vi "Extract TDMS DAQ Info.vi"(8 "error in (no error)":errorcluster, 10 "TDMS Name Mapping":T1, 11 "TDMS File Path":path) -> (0 "error out":errorcluster, 1 "DAQ Sample Rate":dbl, 2 "DAQ Wfm Map":map{string, digitalwaveform}(c390), 3 "DAQ Channels":string[](array[string]))   [LabVIEW 2025]
uses:
  Typedef/TDMS Name Mapping.ctl
  <vilib>/Utility/error.llb/Error Cluster From Error Code.vi
  <vilib>/Waveform/DWDTOps.llb/DWDT Boolean Array to Digital.vi
  <vilib>/ErrorRing/Error Ring.xnode
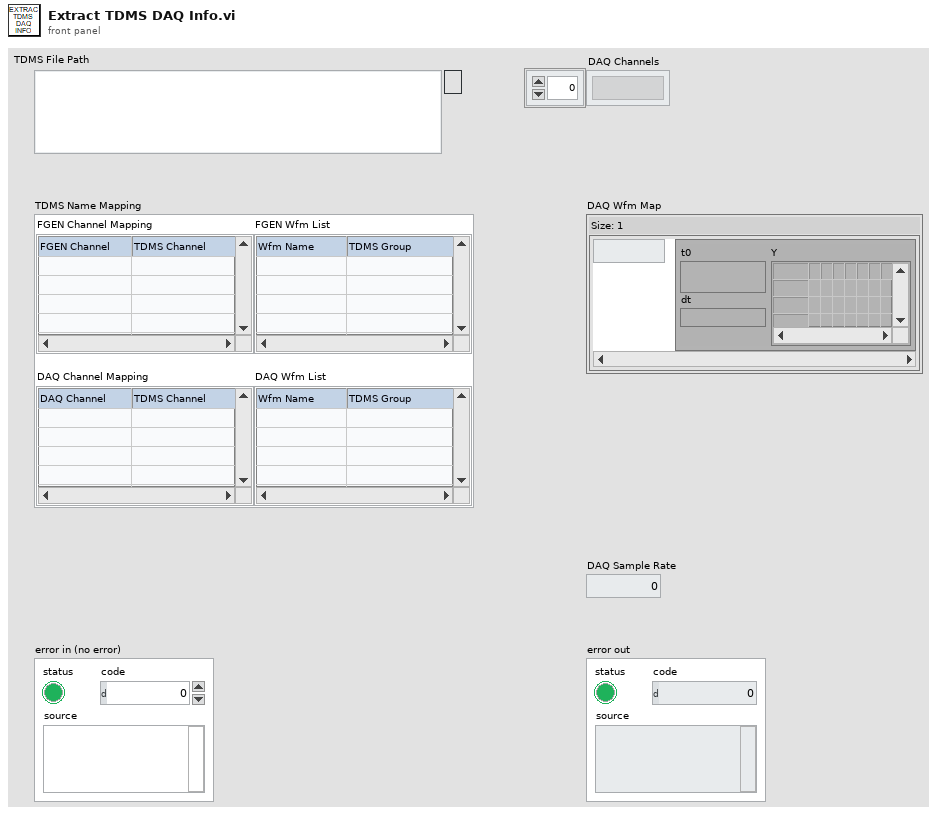
[diagram p1: front panel]
types:
  T1 = typedef "TDMS Name Mapping.ctl" = cluster{"FGEN Channel Mapping":string[][], "DAQ Channel Mapping":string[][], "FGEN Wfm List":string[][], "DAQ Wfm List":string[][]}
  T2 = enum16{"open", "open or create", "create or replace", "create", "open (read-only)"}
  T3 = enum16{"Error or Wfm Not Found", "Not all Chns Found", "All Found"}
  T4 = cluster{"Waveforms":waveform(dbl)[], "Markers":i32}
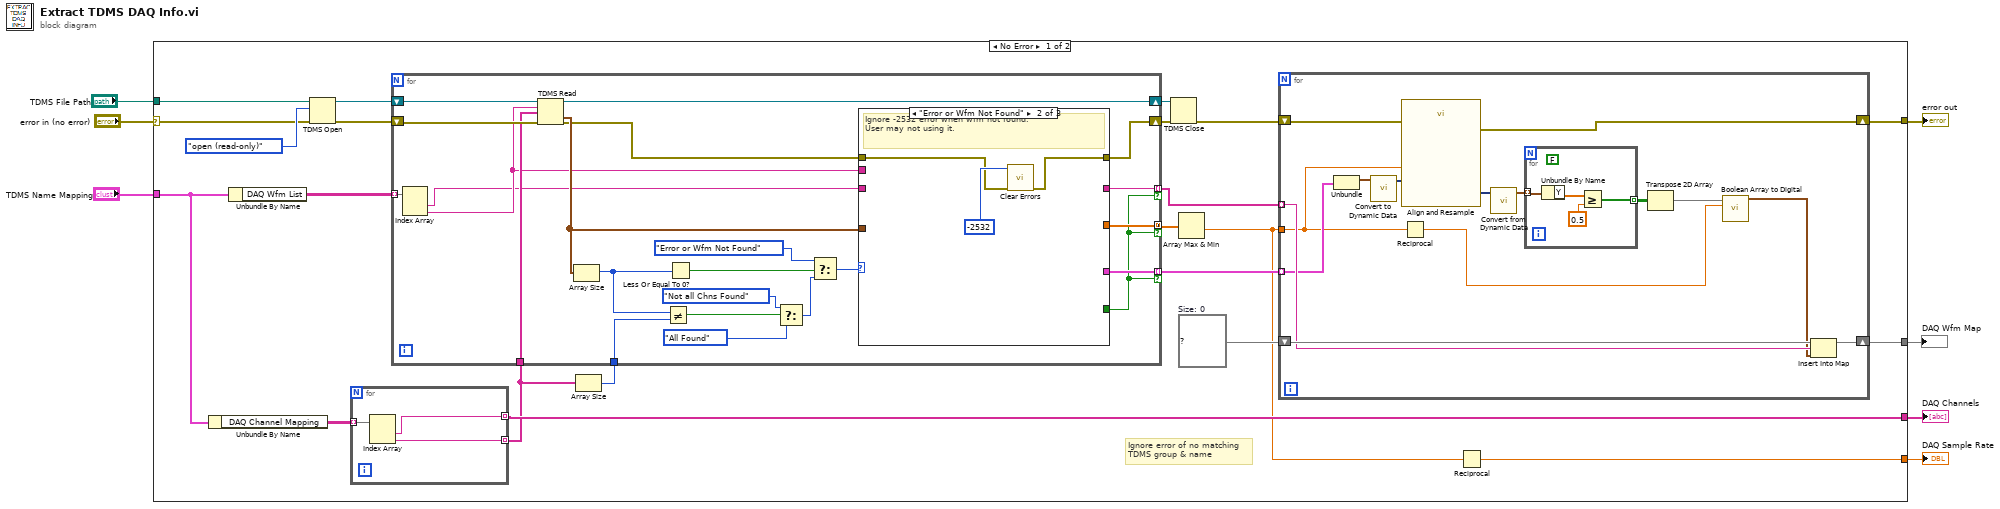
[diagram p0: block diagram]
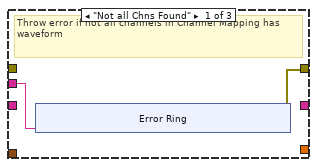
[diagram p2: hidden frame]
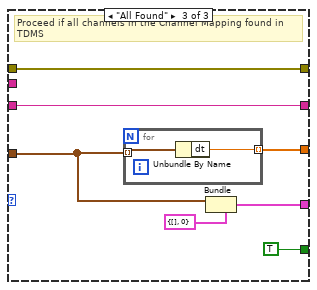
[diagram p3: hidden frame]
diagram:
  n1 = case shown="No Error" "error in (no error)" {
    selector: "error in (no error)" -> [w20 w96]
    tunnel: "TDMS File Path" -> [w27 _]
    tunnel: [w26 _] -> w6
    tunnel: [w14 w96] -> w5
    tunnel: [w13 _] -> w1
    tunnel: [w11 _] -> w3
    tunnel: "TDMS Name Mapping" -> [w10 _]
    frame No Error {
      w17 = map{string, digitalwaveform} {}  # Size: 0
      # "Ignore error of no matching\nTDMS group & name"
      n2 = Unbundle By Name(w10) -> ("DAQ Channel Mapping"=w28:string[][])
      n3 = Unbundle By Name(w10) -> ("DAQ Wfm List"=w29:string[][])
      n4 = TDMS Open(8:w20, 10:T2."open (read-only)" ("operation (0:open)"), 11:w27) -> (0:w24:errorcluster, 3:w25:refnum<k34>)  [unwired: 4 in]
      n5 = for {
        tunnel: w28 -> [w76] mode=indexing
        tunnel: [w75] -> w26 mode=indexing
        tunnel: [w74] -> w9 mode=indexing
        n6 = Index Array(array=w76) -> (element #1=w75:string, element #2=w74:string)  [unwired: 2 in]
      }
      n7 = Array Size(array=w9) -> (size(s)=w8:i32)
      n8 = for {
        tunnel: w29 -> [w52] mode=indexing
        tunnel: [w40] -> w15 mode=indexing if=w39
        tunnel: w9 -> [w46]
        shift-right: [w45] -> w21
        shift-left: w24 -> [w50]
        shift-right: [w49] -> w22
        shift-left: w25 -> [w51]
        tunnel: [w48] -> w18 mode=indexing if=w39
        tunnel: [w47] -> w19 mode=concatenating if=w39
        tunnel: w8 -> [w31]
        n9 = Index Array(array=w52) -> (element #1=w41:string, element #2=w42:string)  [unwired: 2 in]
        n10 = TDMS Read(0:w51, 5:w42, 7:w46, 11:w50) -> (4:w49:refnum<k34>, 10:w44:waveform(dbl)[], 15:w43:errorcluster)  [unwired: 4 in, 3 out]
        n11 = Array Size(array=w44) -> (size(s)=w32:i32)
        n12 = Not Equal?(x=w32, y=w31) -> (x != y?=w34:bool)
        n13 = Less Or Equal To 0?(x=w32) -> (x <= 0?=w37:bool)
        n14 = Select(t=T3."Not all Chns Found", s=w34, f=T3."All Found") -> (s? t:f=w35:T3)
        n15 = Select(t=T3."Error or Wfm Not Found", s=w37, f=w35) -> (s? t:f=w30:T3)
        n16 = case shown="\"Error or Wfm Not Found\"" w30 {
          tunnel: [_ _ w70] -> w48
          tunnel: w44 -> [_ _ w66]
          tunnel: [_ _ w69] -> w47
          tunnel: w43 -> [_ w63 w68]
          tunnel: [w53 w62 w68] -> w45
          tunnel: w42 -> [w54 _ _]
          tunnel: w41 -> [_ _ w67]
          tunnel: [_ _ w67] -> w40
          tunnel: [_ _ TRUE] -> w39
          frame "Not all Chns Found" {
            # "Throw error if not all channels in Channel Mapping has waveform"
            n17 = xnode "Error Ring"("parameter 0"=w54) -> ("error out"=w53:errorcluster)
          }
          frame "Error or Wfm Not Found" {
            # "Ignore -2532 error when wfm not found.\nUser may not using it."
            n18 = call <vilib>:"Clear Errors.vi"("error in (no error)"=w63, "specific error code to clear (0: all)"=-2532) -> ("error out"=w62:errorcluster)  [unwired: 4 in, 1 out]
          }
          frame "All Found" {
            # "Proceed if all channels in the Channel Mapping found in TDMS"
            n19 = for {
              tunnel: w66 -> [w73] mode=indexing
              tunnel: [w72] -> w69 mode=indexing
              n20 = Unbundle By Name(w73) -> ("dt"=w72:dbl)
            }
            n21 = Bundle(cluster=T4 {"Waveforms"=[], "Markers"=0} ("output cluster"), "Waveforms"=w66) -> (w70:T4)  [unwired: 1 in]
          }
        }
      }
      n22 = TDMS Close(8:w21, 11:w22) -> (0:w16:errorcluster)  [unwired: 1 out]
      n23 = Array Max & Min(array=w19) -> (min value=w12:dbl)  [unwired: 3 out]
      n24 = for {
        tunnel: w18 -> [w83] mode=indexing
        shift-right: [w90] -> w13
        shift-left: w17 -> [w91]
        tunnel: w12 -> [w81]
        shift-right: [w88] -> w14
        shift-left: w16 -> [w89]
        tunnel: w15 -> [w84] mode=indexing
        n25 = Unbundle(w83) -> ("Waveforms"=w87:waveform(dbl)[])  [unwired: 1 out]
        n26 = call "Convert to Dynamic Data"("Array of Waveforms"=w87) -> ("Dynamic Data Type"=w86:dynamicdata)  [unwired: 3 in]
        n27 = call "Align and Resample"("dt"=w81, "error in (no error)"=w89, "Signals"=w86) -> ("error out"=w88:errorcluster, "Resampled Signals"=w85:dynamicdata)  [unwired: 6 in, 1 out]
        n28 = Reciprocal(x=w81) -> (1/x=w80:dbl)
        n29 = call "Convert from Dynamic Data"("Dynamic Data Type"=w85) -> ("Array of Waveform"=w82:waveform(dbl)[])  [unwired: 3 in]
        n30 = for {
          tunnel: w82 -> [w95] mode=indexing
          tunnel: [w92] -> w79 mode=indexing
          (unwired) FALSE ("compress digital (T)")
          n31 = Unbundle By Name(w95) -> ("Y"=w94:dbl[])
          n32 = Greater Or Equal?(x=w94, y=0.5) -> (x >= y?=w92:bool[])
        }
        n33 = Transpose 2D Array(2D array=w79) -> (transposed array=w78:bool[][])
        n34 = call-poly <vilib>:"Boolean Array to Digital.vi"("sample rate"=w80, "boolean array"=w78) -> ("digital waveform"=w77:digitalwaveform)  [unwired: 8 in, 1 out]
        n35 = Insert Into Map(map in=w91, key=w84, value=w77) -> (map out=w90:map{string, digitalwaveform})  [unwired: 2 out]
      }
      n36 = Reciprocal(x=w12) -> (1/x=w11:dbl)
    }
    frame Error {
    }
  }
  "DAQ Channels" <- w6
  "error out" <- w5
  "DAQ Sample Rate" <- w3
  "DAQ Wfm Map" <- w1
